vi "Set Title.vi"() -> (0 "error out":errorcluster)   [LabVIEW 2017]
panel:
  out "n":i32
  out "i":i32
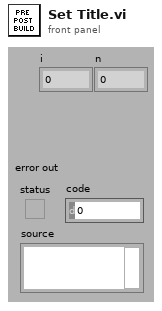
[diagram p1: front panel]
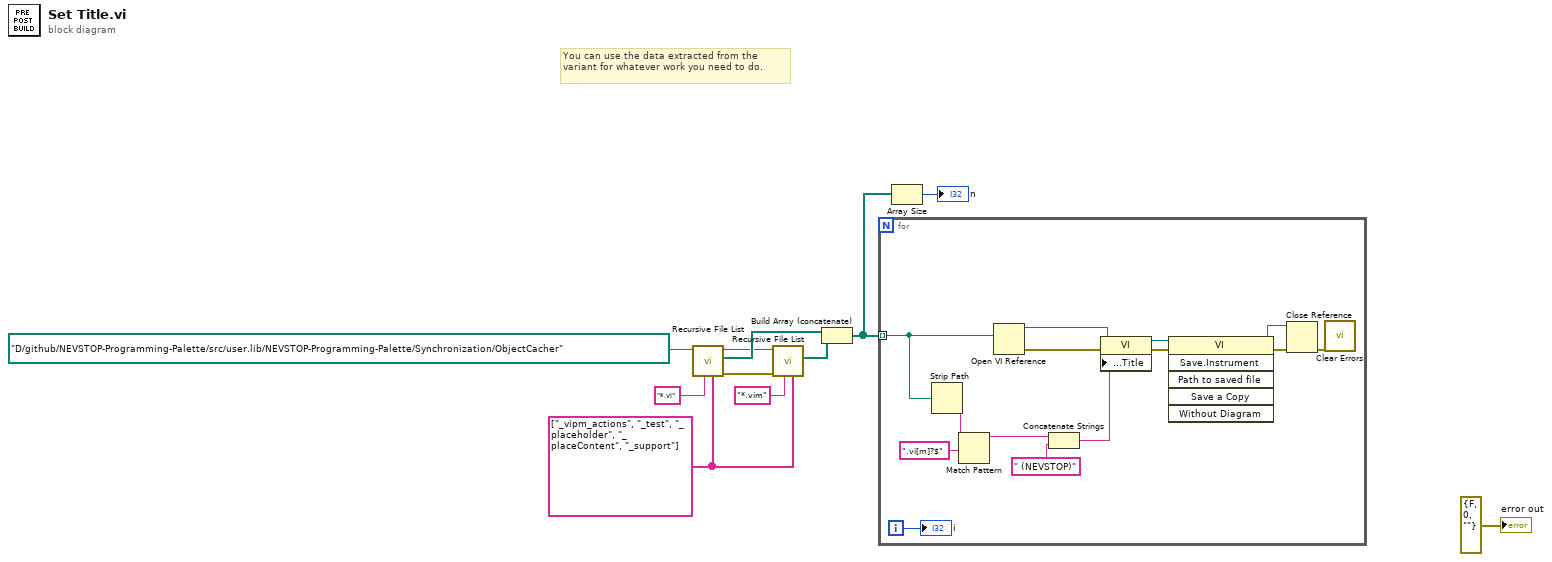
[diagram p0: block diagram]
diagram:
  w3 = string[] ["_vipm_actions", "_test", "_placeholder", "_placeContent", "_support"] ("Folders to Exclude")
  # "You can use the data extracted from the variant for whatever work you need to do."
  n1 = call <vilib>:"Recursive File List.vi"("Folders to Exclude"=w3, "pattern"="*.vi", "Folder Path"=path "D:/github/NEVSTOP-Programming-Palette/src/user.lib/NEVSTOP-Programming-Palette/Synchronization/ObjectCacher") -> ("error out"=w8:errorcluster, "All Files in Dir"=w7:path[], "dup Folder Path"=w4:path)  [unwired: 4 in, 2 out]
  n2 = call <vilib>:"Recursive File List.vi"("Folders to Exclude"=w3, "pattern"="*.vim", "error in (no error)"=w8, "Folder Path"=w4) -> ("All Files in Dir"=w6:path[])  [unwired: 3 in, 4 out]
  n3 = Build Array (concatenate)(w7, w6) -> (w2:path[])
  n4 = for {
    tunnel: w2 -> [w19] mode=indexing
    i -> [w13]
    n5 = Strip Path(path=w19) -> (name=w18:string)  [unwired: 1 out]
    n6 = Match Pattern(string=w18, regular expression=".vi[m]?$") -> (before substring=w16:string)  [unwired: 1 in, 3 out]
    n7 = Open VI Reference(vi path=w19) -> (vi reference=w25:refnum<vi>, error out=w20:errorcluster)  [unwired: 5 in]
    n8 = Concatenate Strings(w16, " (NEVSTOP)" ("string")) -> (w15:string)
    n9 = property class="VI"(reference=w25, error in=w20, "Front Panel.Title"=w15) -> (reference out=w24:refnum<vi>, error out=w23:errorcluster)
    n10 = invoke class="VI" method="Save.Instrument"(reference=w24, error in=w23) -> (reference out=w21:refnum<vi>, error out=w22:errorcluster)  [unwired: 4 in, 4 out]
    n11 = Close Reference(reference=w21, error in (no error)=w22) -> (error out=w12:errorcluster)
    n12 = call <vilib>:"Clear Errors.vi"("error in (no error)"=w12) -> ()  [unwired: 5 in, 2 out]
    "i" <- w13
  }
  n13 = Array Size(array=w2) -> (size(s)=→"n":i32)
  "error out" <- errorcluster {"status"=FALSE, "code"=0, "source"=""} ("error out")
